vi "Update VS channels (object info).vi"(9 "reflectAttributeValues in":T1, 10 "hla map helpers in":T6, 11 "values in":dbl[](array[numeric])) -> (1 "reflectAttributeValues out":T1, 2 "hla map helpers out":T6, 3 "values out":dbl[](array[numeric]))   [LabVIEW 2019, in "HLA Custom Device Engine.lvlib"]
uses:
  HLA Custom Device Engine.lvlib
  _typedefs/RThlaMapHelpers.ctl
  _typedefs/map_interaction.ctl
  _typedefs/map_interaction_value.ctl
  _typedefs/map_attr_param_data.ctl
  _typedefs/map_object.ctl
  _typedefs/map_object_key.ctl
  _typedefs/map_object_value.ctl
  _typedefs/map_object_instance.ctl
  _typedefs/map_object_instance_value.ctl
  _typedefs/map_object_vs_instance.ctl
  _typedefs/reflectAttributeValues_type.ctl
  _typedefs/object_info_received_type.ctl
  emea-ni-adg-hla-lv/src/library/typedefs/TransportationType.ctl
  emea-ni-adg-hla-lv/src/library/typedefs/OrderType.ctl
  _typedefs/dataElement_type.ctl
  emea-ni-adg-hla-lv/src/library/openrti_rti1516eLv.lvlib
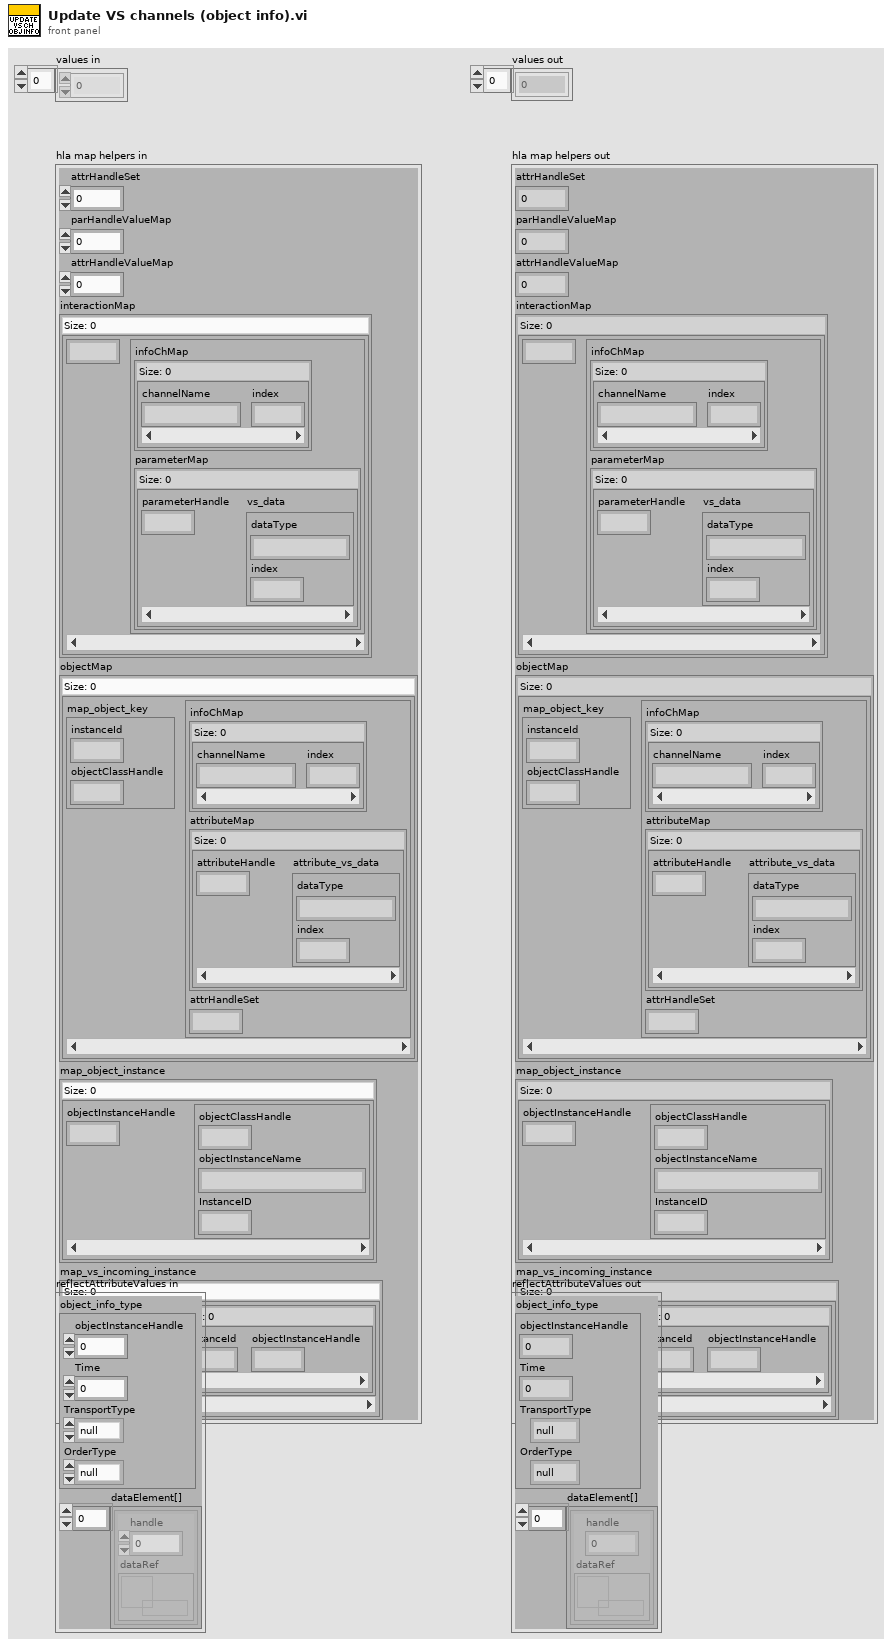
[diagram p1: front panel]
types:
  T1 = typedef "HLA Custom Device Engine.lvlib/reflectAttributeValues_type.ctl" = cluster{"object_info_type":T2, "dataElement[]":T5[]}
  T2 = typedef "HLA Custom Device Engine.lvlib/object_info_received_type.ctl" = cluster{"objectInstanceHandle":u64, "Time":u32, "TransportType":T3, "OrderType":T4}
  T3 = typedef "openrti_rti1516eLv.lvlib/TransportationType.ctl" = enum32{"null", "RELIABLE", "BEST_EFFORT"}
  T4 = typedef "openrti_rti1516eLv.lvlib/OrderType.ctl" = enum32{"null", "RECEIVE", "TIMESTAMP"}
  T5 = typedef "HLA Custom Device Engine.lvlib/dataElement_type.ctl" = cluster{"handle":u64, "dataRef":refnum<data-value>}
  T6 = typedef "HLA Custom Device Engine.lvlib/RThlaMapHelpers.ctl" = cluster{"attrHandleSet":u64, "parHandleValueMap":u64, "attrHandleValueMap":u64, "interactionMap":T7, "objectMap":T10, "map_object_instance":T13, "map_vs_incoming_instance":T15}
  T7 = typedef "HLA Custom Device Engine.lvlib/map_interaction.ctl" = map{u64, T8}
  T8 = typedef "HLA Custom Device Engine.lvlib/map_interaction_value.ctl" = cluster{"infoChMap":map{string, i32}, "parameterMap":map{u64, T9}}
  T9 = typedef "HLA Custom Device Engine.lvlib/map_attr_param_data.ctl" = cluster{"dataType":string, "index":i32}
  T10 = typedef "HLA Custom Device Engine.lvlib/map_object.ctl" = map{T11, T12}
  T11 = typedef "HLA Custom Device Engine.lvlib/map_object_key.ctl" = cluster{"instanceId":i32, "objectClassHandle":u64}
  T12 = typedef "HLA Custom Device Engine.lvlib/map_object_value.ctl" = cluster{"infoChMap":map{string, i32}, "attributeMap":map{u64, T9}, "attrHandleSet":u64}
  T13 = typedef "HLA Custom Device Engine.lvlib/map_object_instance.ctl" = map{u64, T14}
  T14 = typedef "HLA Custom Device Engine.lvlib/map_object_instance_value.ctl" = cluster{"objectClassHandle":u64, "objectInstanceName":string, "InstanceID":i32}
  T15 = typedef "HLA Custom Device Engine.lvlib/map_object_vs_instance.ctl" = map{u64, map{i32, u64}}
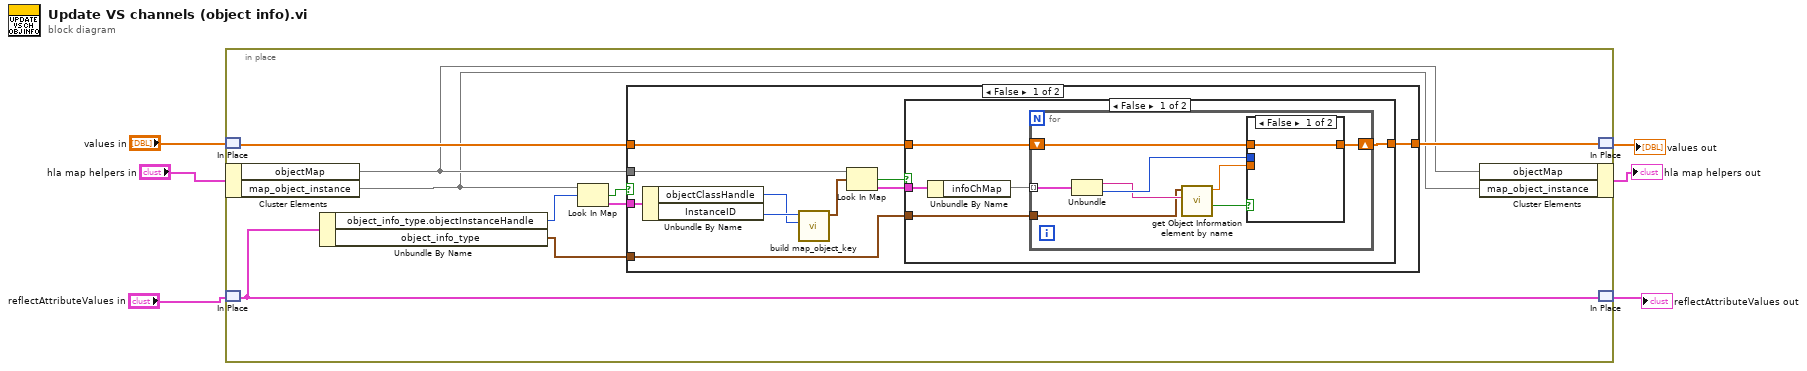
[diagram p0: block diagram]
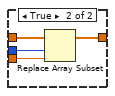
[diagram p2: hidden frame]
diagram:
  n1 = in-place {
    n2 = in-place-match #1("values in") -> (w15:dbl[])
    n3 = in-place-cluster #2("hla map helpers in") -> ("objectMap"=w13:T10, "map_object_instance"=w10:T13)
    n4 = in-place-match #3("reflectAttributeValues in") -> (w12:T1)
    n5 = Unbundle By Name(w12) -> ("object_info_type.objectInstanceHandle"=w11:u64, "object_info_type"=w7:T2)
    n6 = Look In Map(map=w10, key=w11) -> (key not found?=w9:bool, value=w8:T14)  [unwired: 1 in]
    n7 = case shown="False" w9 {
      tunnel: w15 -> [w23 w45]
      tunnel: [w22 w45] -> w14
      tunnel: w13 -> [w21 _]
      tunnel: w7 -> [w20 _]
      tunnel: w8 -> [w19 _]
      frame False {
        n8 = Unbundle By Name(w19) -> ("objectClassHandle"=w16:u64, "InstanceID"=w17:i32)
        n9 = call "build map_object_key.vi"("objectClassHandle"=w16, "instanceId"=w17) -> ("object_map_key"=w18:T11)  [unwired: 9 in]
        n10 = Look In Map(map=w21, key=w18) -> (key not found?=w25:bool, value=w24:T12)  [unwired: 1 in]
        n11 = case shown="False" w25 {
          tunnel: [w29 w44] -> w22
          tunnel: w24 -> [w27 _]
          tunnel: w23 -> [w28 w44]
          tunnel: w20 -> [w26 _]
          frame False {
            n12 = Unbundle By Name(w27) -> ("infoChMap"=w30:map{string, i32})
            n13 = for {
              tunnel: w30 -> [w33] mode=indexing
              shift-right: [w37] -> w29
              shift-left: w28 -> [w38]
              tunnel: w26 -> [w31]
              n14 = Unbundle(w33) -> ("channelName"=w32:string, "index"=w35:i32)
              n15 = call "get Object Information element by name.vi"("name"=w32, "interaction_attribute_type"=w31) -> ("found"=w34:bool, "element out"=w36:dbl)  [unwired: 8 in]
              n16 = case shown="False" w34 {
                tunnel: w38 -> [w39 w43]
                tunnel: [w39 w42] -> w37
                tunnel: w36 -> [_ w41]
                tunnel: w35 -> [_ w40]
                frame False {
                }
                frame True {
                  n17 = Replace Array Subset(array=w43, new element=w41, index=w40) -> (w42:dbl[])
                }
              }
            }
          }
          frame True {
          }
        }
      }
      frame True {
      }
    }
    n18 = in-place-cluster #2("objectMap"=w13, "map_object_instance"=w10) -> (→"hla map helpers out":T6)
    n19 = in-place-match #1(w14) -> (→"values out":dbl[])
    n20 = in-place-match #3(w12) -> (→"reflectAttributeValues out":T1)
  }
